vi "ReversedEngineering StateReverseDialog.vi"(5 "error in (no error)":errorcluster, 6 "NewDiagram":bool) -> (15 "StateDiagramReverseOptions":T5={"Clear All Current States"=FALSE, "UseMenuItem"=TRUE, "InsertArrayQueuedElementsVI"="", "Add Actions"=TRUE, "StateDiagramSerachActions"={"Action"=enum."OnlyTheseVIs", "VINames"=[], "LimitActions(VIs)"=0}, "AddCaseCommentsAsActions"=FALSE, "IgnoreStatesNotUsed"=FALSE, "CommentsSerachActions"={"MinimumTextLength"=0, "OnlyTopLeftComment"=FALSE, "CommentPrefix"=""}, "TransitionMode"=enum."Add to current transtion text", "ActionMode"=enum."Add to current action text"}, 16 "Cancel":bool, 19 "error out":errorcluster)   [LabVIEW 2012]
uses:
  <resource>/Framework/Providers/Open_GDS/UML/ReversedEngineering/private/ReversedEngineering StateDiagramReverseOptions.ctl
  <resource>/Framework/Providers/Open_GDS/UML/ReversedEngineering/private/ReversedEngineering StateDiagramSerachActions.ctl
  <resource>/Framework/Providers/Open_GDS/UML/ReversedEngineering/ReversedEngineering StateAnalyseVIAction.ctl
  <resource>/Framework/Providers/Open_GDS/UML/ReversedEngineering/private/ReversedEngineering StateDiagramCommentSearchType.ctl
  <resource>/Framework/Providers/Open_GDS/UML/UMLEditor/UMLEditor_StoredPathes.ctl
  <resource>/Framework/Providers/Open_GDS/UML/ContextHelp/ContextHelp_HelpTexts.ctl
  <resource>/Framework/Providers/Open_GDS/ClassProviders/Common/File/File_StoredPathesActions.ctl
panel:
  in  "ActionMode":T1(ring) caption="Action text"
  in  "TransitionMode":T2(ring) caption="Transition text"
  in  "CommentsSerachActions":T3
  in  "IgnoreStatesNotUsed":bool caption="Using Queued Based State Machines"
  in  "AddCaseCommentsAsActions":bool caption="Using Queued Based State Machines"
  in  "QueuedSettings":bool
  in  "UseQueuedStateMachines":bool caption="Using Queued Based State Machines"
  in  "Help":bool
  in  "SearchCriteria":T4={"NoOfAction"=10, "VI-List"=[], "VI-filter"=0, "ClearList"=FALSE, "AddVI"=FALSE, "AddVIs"=FALSE, "AddVIsRec"=FALSE} caption="Search for Actions(VIs)" {"VI-filter" items=["<Do not use VI-filter>", "Only allow VI-s found in the VI-List", "Allow all VIs except the ones in the VI-List"]; "NoOfAction" min=1 max=50}
  in  "SearchForVIs":bool
  in  "Cancel":bool
  in  "OK":bool
  in  "ClearStates":bool caption="Clear All Current States on the diagram"
  # "If the states should be search it checks all subvis and functions in every case."
  # "Select what actions(functions) that should be searched for. If the selected action exists in the state this action will be listed in the diagram."
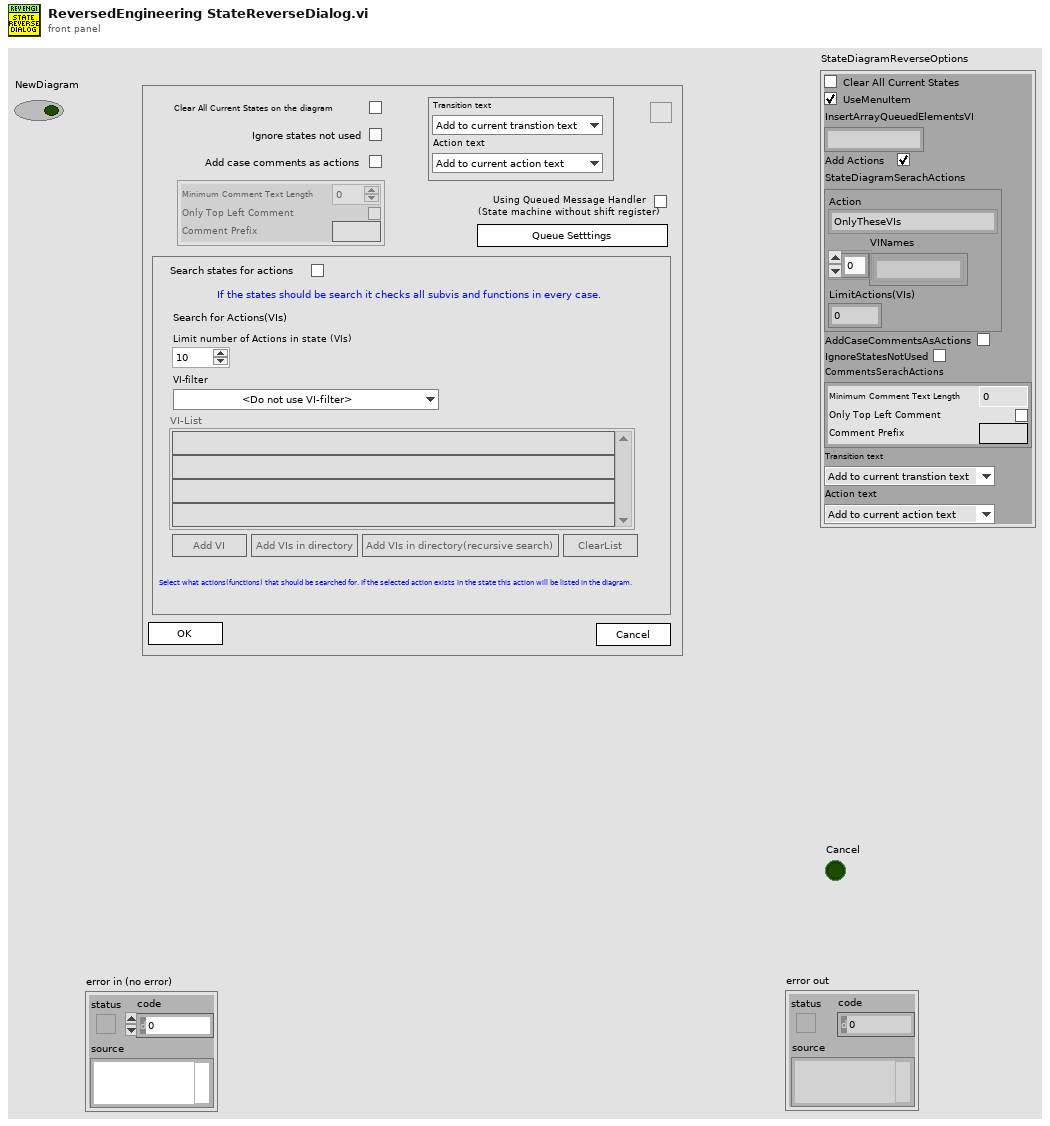
[diagram p1: front panel]
types:
  T1 = enum16{"Add to current action text", "Replace action text"}
  T2 = enum16{"Add to current transtion text", "Replace transition text"}
  T3 = typedef "ReversedEngineering StateDiagramCommentSearchType.ctl" = cluster{"MinimumTextLength":i32, "OnlyTopLeftComment":bool, "CommentPrefix":string}
  T4 = cluster{"NoOfAction":i32, "VI-List":string[], "VI-filter":u16, "ClearList":bool, "AddVI":bool, "AddVIs":bool, "AddVIsRec":bool}
  T5 = typedef "ReversedEngineering StateDiagramReverseOptions.ctl" = cluster{"Clear All Current States":bool, "UseMenuItem":bool, "InsertArrayQueuedElementsVI":string, "Add Actions":bool, "StateDiagramSerachActions":T6, "AddCaseCommentsAsActions":bool, "IgnoreStatesNotUsed":bool, "CommentsSerachActions":T3, "TransitionMode":enum16{"Add to current transtion text", "Replace transition text"}, "ActionMode":enum16{"Add to current action text", "Replace action text"}}
  T6 = typedef "ReversedEngineering StateDiagramSerachActions.ctl" = cluster{"Action":T7, "VINames":string[], "LimitActions(VIs)":i32}
  T7 = typedef "ReversedEngineering StateAnalyseVIAction.ctl" = enum16{"OnlyTheseVIs", "NotTheseVIs"}
  T8 = typedef "UMLEditor_StoredPathes.ctl" = enum16{"LastSearchPath", "QueuedArrayStateVI", "ClassBasePath", "ViTemplatePath", "ApplicationTemplatePath", "IniFilePath", "WizDir", "RevPlugInPath"}
  T9 = typedef "ContextHelp_HelpTexts.ctl" = enum16{"None(Hide)", "Default", "Help", "Welcome", "GettingStarted", "ClassDiagram_Help", "SequenceDiagram_Help", "UseCaseDiagram_Help", "BSelect", "BClass", "BInterface", "BPackage", "BNote", "BDependency", "BInheritance", "BInterfaceImplementation", "BAssociation", "BAggregation", "BCompAggregation", "BNoteConnector", "BObject", "BActionBar", "BCall", "BSystem", "BActor", "BUseCase", "BGeneralization", "BIncludes", "BExtends", "BUseCaseDiagramAssociation", "ClassRelationshipEdge editDialog_Bent Style", "ClassRelationshipEdge editDialog_RelationType", "ClassRelationshipEdge editDialog_Reverse association", "ClassRelationshipEdge editDialog_Start label", "ClassRelationshipEdge editDialog_Middle label", "ClassRelationshipEdge editDialog_End label", "UMLEditor reversedEngineering_Pathes", "ReversedEngineering StateReverseDialog_Help", "ReversedEngineering StateQueuedSettings_Help", "UMLEditor reversedEngineering_AddTopVIs", "UMLEditor reversedEngineering_AddClasses", "UMLEditor reversedEngineering_AddDirs", "UMLEditor reversedEngineering_Recursively", "UMLEditor reversedEngineering_Remove", "UMLEditor reversedEngineering_ClearList", "UMLEditor reversedEngineering_HideSubAss", "UMLEditor reversedEngineering_CreateTypes", "UMLEditor reversedEngineering_OnlyInheritance", "UMLEditor reversedEngineering_CreateApplication", "UMLEditor reversedEngineering_OK", "UMLEditor reversedEngineering_Cancel", "UMLEditor reversedEngineering_Help", "UMLEditor createWizardScriptFile_ScriptfilePath", "UMLEditor createWizardScriptFile_ClassPath", "UMLEditor createWizardScriptFile_Use", "UMLEditor createWizardScriptFile_PrivateDirName", "UMLEditor createWizardScriptFile_DirAppend", "UMLEditor createWizardScriptFile_Separator Character", "UMLEditor createWizardScriptFile_OK", "UMLEditor createWizardScriptFile_Cancel", "UMLEditor createWizardScriptFile_Help", "ClassNode editDialog_Class Name", "InterfaceNode editDialog_Class Name", "ClassNode editDialog_Attribute", "ClassNode editDialog_Methods", "InterfaceNode editDialog_Methods", "ClassNode editDialog_connection", "InterfaceNode editDialog_connection", "ClassNode editDialog_StereoType", "ClassNode editDialog_ShowAttrib", "ClassNode editDialog_ShowMethods", "ClassNode editDialog_ClassPath", "ClassNode editDialog_AddAttribute", "ClassNode editDialog_AddMethod", "InterfaceNode editDialog_AddMethod", "ClassNode AttributeGuide_AttributeName", "ClassNode AttributeGuide_Array?", "ClassNode AttributeGuide_Data Type", "ClassNode AttributeGuide_RefName", "ClassNode AttributeGuide_Preview", "ClassNode AttributeGuide_OK", "ClassNode AttributeGuide_Cancel", "ClassNode MethodGuide_Visibility", "ClassNode MethodGuide_Method Name", "ClassNode MethodGuide_Preview", "ClassNode MethodGuide_OK", "ClassNode MethodGuide_Cancel", "CallNode EditCallProperties_AllButtons", "ObjectNode EditObjectlProperties_AllButtons", "ActorNode EditActorProperties_AllButtons", "UseCaseRelationshipNode EditUseCaselProperties_AllButtons", "UseCaseNode EditUseCaselProperties_AllButtons", "SystemNode EditSystemProperties_AllButtons", "ReversedEngineering UpdateAttributes_AllButtons", "StateNode editDialog_AllButtons", "StateTransition editDialog_AllButtons", "ArrangeNodes Main_Picture", "ArrangeNodes Main_Zoom", "ArrangeNodes Main_Auto Zoom", "ArrangeNodes Main_shorten", "ArrangeNodes Main_Min Length", "ArrangeNodes Main_Max Length", "ArrangeNodes Main_increase", "ArrangeNodes Main_decrease", "ArrangeNodes Main_Shake", "ArrangeNodes Main", "BState", "BInitialState", "BFinalState", "BStateTransition", "StateDiagram_Help", "StateDiagram_PropertiesAllButtons", "ReversedEngineering StateReverseDialog_ClearStates", "ReversedEngineering StateReverseDialog_UseQueuedStateMachines", "ReversedEngineering StateReverseDialog_QueuedSettings", "ReversedEngineering StateReverseDialog_SearchForVIs", "ReversedEngineering StateReverseDialog_SearchCriteria", "OptionsDialog_ClassBasePath", "OptionsDialog_VIPath", "OptionsDialog_ApplicationPath", "OptionsDialog_WizDir", "OptionsDialog_IniFilePath", "OptionsDialog_DefineColors", "OptionsDialog_Help", "OptionsDialog_CreateTypes", "ClassRelationshipEdge editDialog_SplitWire"}
  T10 = typedef "File_StoredPathesActions.ctl" = enum16{"Get Path", "Set Path", "Delete Path", "Clear All Paths"}
  T11 = typedef "ContextHelp_ShowType.ctl" = cluster{"Header":string, "Picture":picture, "Text":string}
  T12 = enum32{"existing file", "new file", "new or existing file", "existing dir", "new dir", "new or existing dir", "existing file (use LLBs)", "new file (use LLBs)", "new or existing file (use LLBs)", "new or existing file or directory (use LLBs)"}
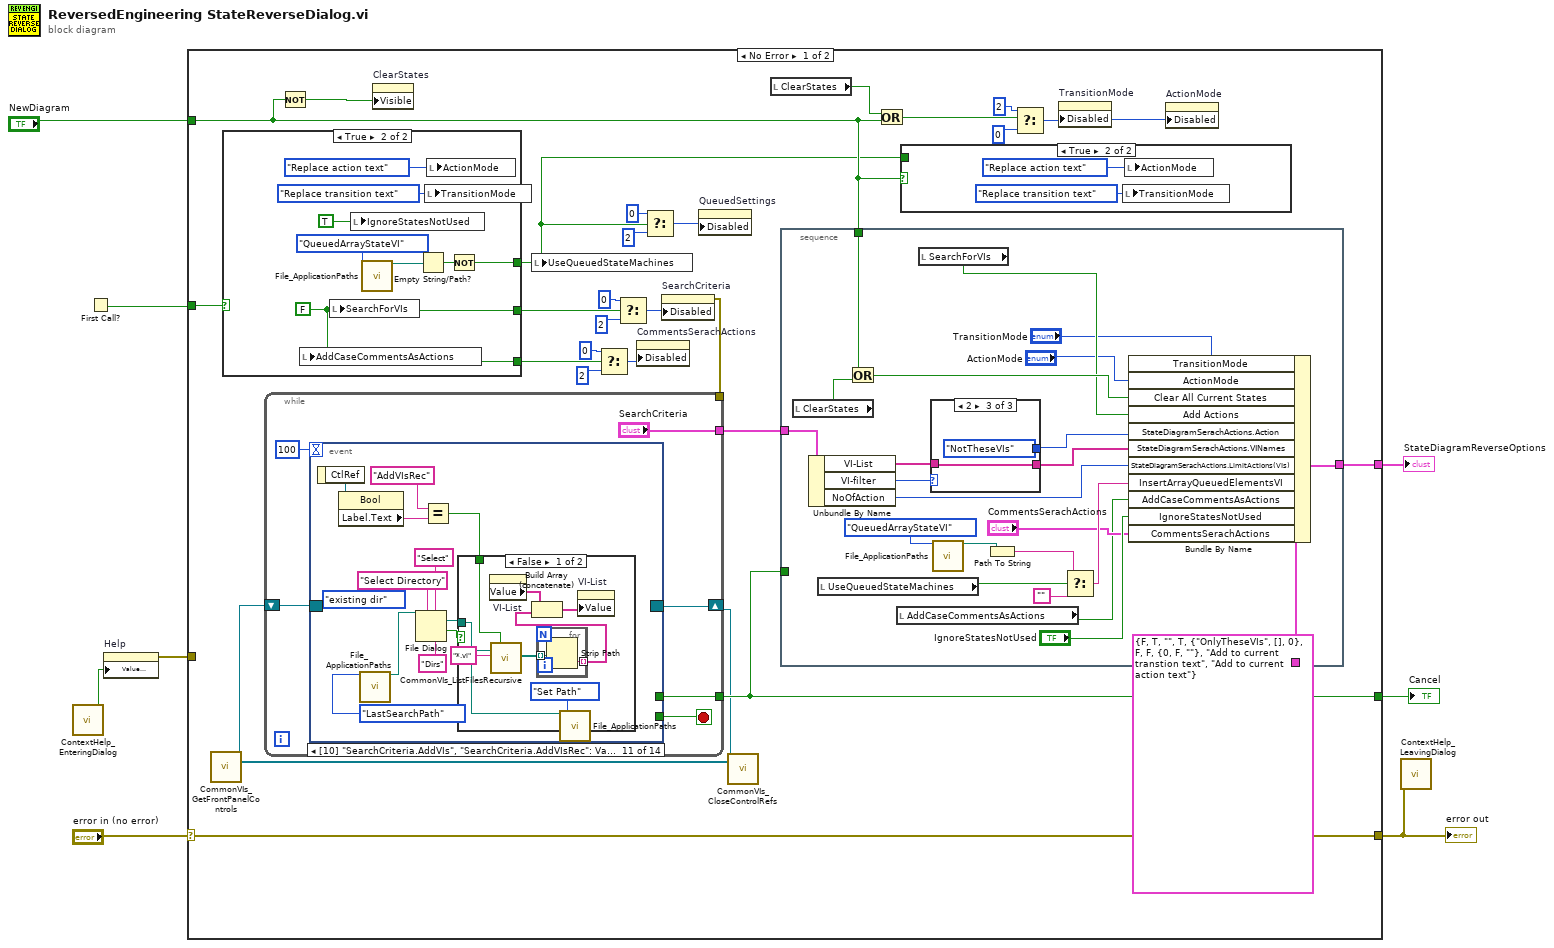
[diagram p0: block diagram]
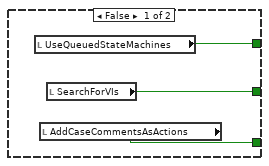
[diagram p3: hidden frame]
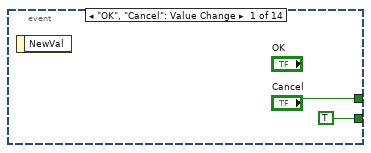
[diagram p4: hidden frame]
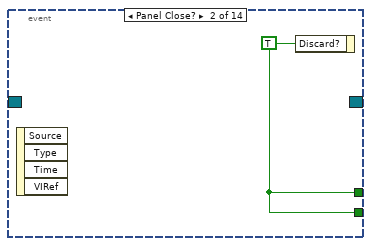
[diagram p5: hidden frame]
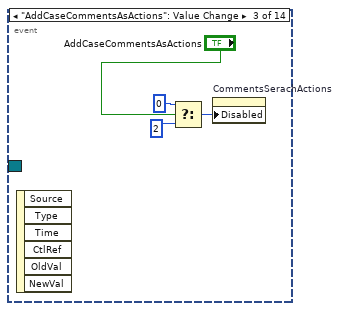
[diagram p6: hidden frame]
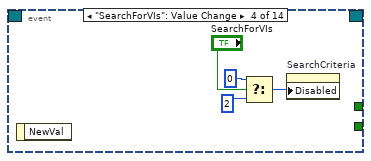
[diagram p7: hidden frame]
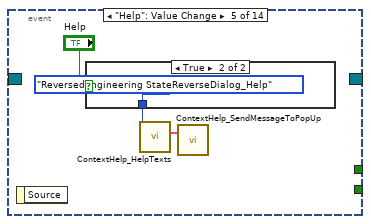
[diagram p8: hidden frame]
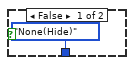
[diagram p9: hidden frame]
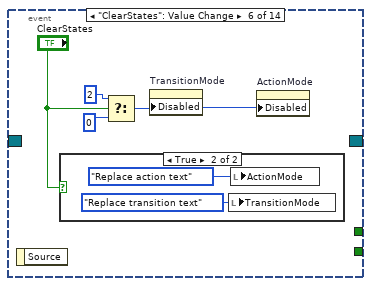
[diagram p10: hidden frame]
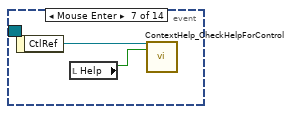
[diagram p12: hidden frame]
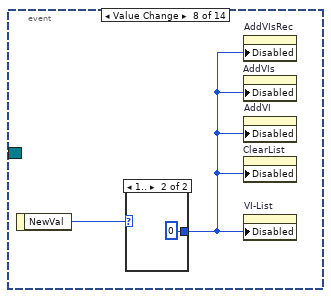
[diagram p13: hidden frame]
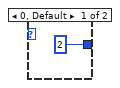
[diagram p14: hidden frame]
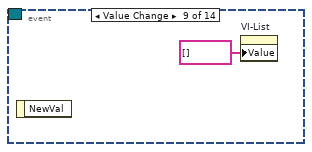
[diagram p15: hidden frame]
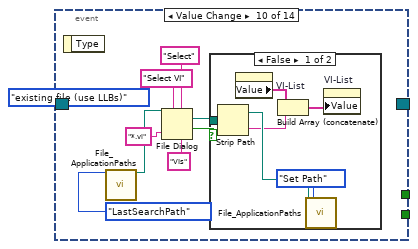
[diagram p16: hidden frame]
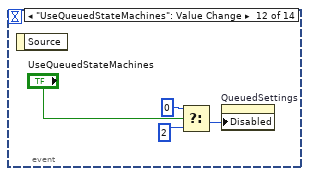
[diagram p19: hidden frame]
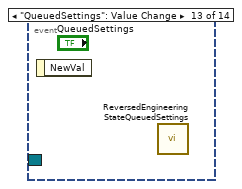
[diagram p20: hidden frame]
diagram:
  n1 = call <resource>:"ContextHelp_EnteringDialog.vi"() -> ("HelpStatus"=w4:bool)  [unwired: 1 in, 18 out]
  n2 = First Call?() -> (First Call?: T/F=w1:bool)
  n3 = property on="Help" class="Bool (strict)"("Value (Signaling)"=w4) -> (error out=w3:errorcluster)  [unwired: 2 in, 1 out]
  n4 = case shown="No Error" "error in (no error)" {
    selector: "error in (no error)" -> [w35 w155]
    tunnel: [w35 w155] -> w2
    tunnel: [w34 _] -> w7
    tunnel: [w36 _] -> w6
    tunnel: "NewDiagram" -> [w10 _]
    tunnel: w3 -> [_ _]
    tunnel: w1 -> [w27 _]
    frame No Error {
      n5 = call <resource>:"CommonVIs_GetFrontPanelControls.vi"() -> ("Event Registration Refnum"=w25:refnum<event-registration>, "ControlRefs"=w23:refnum<vi>[])  [unwired: 2 in, 16 out]
      n6 = case shown="True" w27 {
        tunnel: [w42 w46] -> w26
        tunnel: [w41 w47] -> w9
        tunnel: [w40 w46] -> w16
        frame False {
          n7 = local read "UseQueuedStateMachines"() -> (w41:bool)
          n8 = local read "AddCaseCommentsAsActions"() -> (w40:bool)
          n9 = local read "SearchForVIs"() -> (w42:bool)
        }
        frame True {
          w46 = FALSE ("SearchForVIs")
          n10 = local write "AddCaseCommentsAsActions"(w46) -> ()
          n11 = local write "SearchForVIs"(w46) -> ()
          n12 = local write "IgnoreStatesNotUsed"(TRUE ("IgnoreStatesNotUsed")) -> ()
          n13 = call <resource>:"File_ApplicationPaths.vi"("PathName"=UMLEditor_StoredPathes."QueuedArrayStateVI" ("UMLPathes")) -> ("Path Out"=w49:path)  [unwired: 3 in, 15 out]
          n14 = Empty String/Path?(string/path=w49) -> (empty?=w48:bool)
          n15 = local write "TransitionMode"(T2."Replace transition text" ("TransitionMode")) -> ()
          n16 = local write "ActionMode"(T1."Replace action text" ("ActionMode")) -> ()
          n17 = Not(x=w48) -> (.not. x?=w47:bool)
        }
      }
      n18 = Not(x=w10) -> (.not. x?=w29:bool)
      n19 = property on="ClearStates" class="Bool (strict)"("Visible"=w29) -> ()  [unwired: 2 in, 2 out]
      n20 = local write "UseQueuedStateMachines"(w9) -> ()
      n21 = Select(t=u8 0, s=w16, f=u8 2 ("Disabled")) -> (s? t:f=w17:u8)
      n22 = Select(t=u8 0, s=w26, f=u8 2 ("Disabled")) -> (s? t:f=w31:u8)
      n23 = property on="CommentsSerachActions" class="Clust (strict)"("Disabled"=w17) -> ()  [unwired: 2 in, 2 out]
      n24 = Select(t=u8 0, s=w9, f=u8 2 ("Disabled")) -> (s? t:f=w20:u8)
      n25 = property on="SearchCriteria" class="Clust"("Disabled"=w31) -> (error out=w30:errorcluster)  [unwired: 2 in, 1 out]
      n26 = while {
        tunnel: [w56] -> w34
        tunnel: w30 -> [_]
        tunnel: ["SearchCriteria"] -> w28
        shift-right: [w51] -> w24
        shift-left: w25 -> [w52]
        stop <- w55 stop-if-true
        n27 = event shown="[10] \"SearchCriteria.AddVIs\", \"SearchCriteria.AddVIsRec\": Value Change" {
          selector: w52 -> [_ _ _ _ _ _ _ _ _ _ _ _ _ _]
          dyn-events: [_ _ _ _ _ _ _ _ _ _ _ _ _ _] -> w51
          timeout: 100 -> [_ _ _ _ _ _ _ _ _ _ _ _ _ _]
          tunnel: ["Cancel" w59 _ _ _ _ _ _ _ _ _ _ _ _] -> w56
          tunnel: [TRUE w59 _ _ _ _ _ _ _ _ _ _ _ _] -> w55
          event "OK", "Cancel": Value Change {
            n28 = event-data() -> ()  [unwired: 2 out]
          }
          event Panel Close? {
            w59 = TRUE ("Discard?")
            n29 = event-data() -> ()  [unwired: 5 out]
            n30 = event-data("Discard?"=w59) -> ()  [unwired: 1 in, 1 out]
          }
          event "AddCaseCommentsAsActions": Value Change {
            n31 = event-data() -> ()  [unwired: 7 out]
            n32 = Select(t=u8 0, s="AddCaseCommentsAsActions", f=u8 2 ("Disabled")) -> (s? t:f=w63:u8)
            n33 = property on="CommentsSerachActions" class="Clust (strict)"("Disabled"=w63) -> ()  [unwired: 2 in, 2 out]
          }
          event "SearchForVIs": Value Change {
            n34 = event-data() -> ()  [unwired: 2 out]
            n35 = Select(t=u8 0, s="SearchForVIs", f=u8 2 ("Disabled")) -> (s? t:f=w65:u8)
            n36 = property on="SearchCriteria" class="Clust"("Disabled"=w65) -> ()  [unwired: 2 in, 2 out]
          }
          event "Help": Value Change {
            n37 = event-data() -> ()  [unwired: 2 out]
            n38 = case shown="True" "Help" {
              tunnel: [ContextHelp_HelpTexts."None(Hide)" ("HelpText") ContextHelp_HelpTexts."ReversedEngineering StateReverseDialog_Help" ("HelpText")] -> w69
              frame False {
              }
              frame True {
              }
            }
            n39 = call <resource>:"ContextHelp_HelpTexts.vi"("HelpText (enum or string)"=w69) -> ("HelpOut"=w70:T11)  [unwired: 18 out]
            n40 = call <resource>:"ContextHelp_SendMessageToPopUp.vi"("PopUpMessage"=w70) -> ()  [unwired: 2 in, 17 out]
          }
          event "ClearStates": Value Change {
            n41 = event-data() -> ()  [unwired: 2 out]
            n42 = case shown="True" "ClearStates" {
              frame False {
              }
              frame True {
                n43 = local write "TransitionMode"(T2."Replace transition text" ("TransitionMode")) -> ()
                n44 = local write "ActionMode"(T1."Replace action text" ("ActionMode")) -> ()
              }
            }
            n45 = Select(t=u8 2, s="ClearStates", f=u8 0 ("Disabled")) -> (s? t:f=w76:u8)
            n46 = property on="TransitionMode" class="Enum (strict)"("Disabled"=w76) -> ()  [unwired: 2 in, 2 out]
            n47 = property on="ActionMode" class="Enum (strict)"("Disabled"=w76) -> ()  [unwired: 2 in, 2 out]
          }
          event Mouse Enter {
            n48 = event-data() -> ("CtlRef"=w80:refnum<vi>)  [unwired: 1 out]
            n49 = local read "Help"() -> (w79:bool)
            n50 = call <resource>:"ContextHelp_CheckHelpForControl.vi"("Ctl Refnum"=w80, "Help"=w79) -> ()  [unwired: 1 in, 17 out]
          }
          event "SearchCriteria.VI-filter": Value Change {
            n51 = event-data() -> ("NewVal"=w82:u16)  [unwired: 1 out]
            n52 = case shown="1.." w82 {
              tunnel: [u8 2 ("Disabled") u8 0 ("Disabled")] -> w81
              frame 0, Default {
              }
              frame 1.. {
              }
            }
            n53 = property on="AddVIsRec" class="Bool"("Disabled"=w81) -> ()  [unwired: 2 in, 2 out]
            n54 = property on="AddVIs" class="Bool"("Disabled"=w81) -> ()  [unwired: 2 in, 2 out]
            n55 = property on="AddVI" class="Bool"("Disabled"=w81) -> ()  [unwired: 2 in, 2 out]
            n56 = property on="ClearList" class="Bool"("Disabled"=w81) -> ()  [unwired: 2 in, 2 out]
            n57 = property on="VI-List" class="Arr (strict)"("Disabled"=w81) -> ()  [unwired: 2 in, 2 out]
          }
          event "SearchCriteria.ClearList": Value Change {
            n58 = event-data() -> ()  [unwired: 2 out]
            n59 = property on="VI-List" class="Arr (strict)"("Value"=string[] []) -> ()  [unwired: 2 in, 2 out]
          }
          event "SearchCriteria.AddVI": Value Change {
            (unwired) T12."existing file (use LLBs)" ("select mode (2)")
            n60 = event-data() -> ()  [unwired: 2 out]
            n61 = call <resource>:"File_ApplicationPaths.vi"("PathName"=UMLEditor_StoredPathes."LastSearchPath" ("UMLPathes")) -> ("Path Out"=w91:path)  [unwired: 3 in, 15 out]
            n62 = File Dialog(4:"VIs" ("pattern label"), 5:"Select" ("button label"), 6:"*.vi" ("pattern"), 7:"Select VI" ("prompt"), 11:w91) -> (1:w86:bool, 3:w90:path)  [unwired: 1 in, 3 out]
            n63 = case shown="False" w86 {
              tunnel: w90 -> [w98 _]
              frame False {
                n64 = Strip Path(path=w98) -> (stripped path=w97:path, name=w95:string)
                n65 = property on="VI-List" class="Arr (strict)"() -> ("Value"=w96:string[])  [unwired: 2 in, 2 out]
                n66 = Build Array (concatenate)(w96, w95) -> (w94:string[])
                n67 = call <resource>:"File_ApplicationPaths.vi"("Path In"=w97, "Method (Get Path)"=File_StoredPathesActions."Set Path") -> ()  [unwired: 2 in, 16 out]
                n68 = property on="VI-List" class="Arr (strict)"("Value"=w94) -> ()  [unwired: 2 in, 2 out]
              }
              frame True {
              }
            }
          }
          event "SearchCriteria.AddVIs", "SearchCriteria.AddVIsRec": Value Change {
            (unwired) T12."existing dir" ("select mode (2)")
            n69 = event-data() -> ("CtlRef"=w103:refnum<vi>)  [unwired: 1 out]
            n70 = property class="Bool"(reference=w103) -> ("Label.Text"=w102:string)  [unwired: 1 in, 2 out]
            n71 = call <resource>:"File_ApplicationPaths.vi"("PathName"=UMLEditor_StoredPathes."LastSearchPath" ("UMLPathes")) -> ("Path Out"=w108:path)  [unwired: 3 in, 15 out]
            n72 = File Dialog(4:"Dirs" ("pattern label"), 5:"Select" ("button label"), 7:"Select Directory" ("prompt"), 11:w108) -> (1:w104:bool, 3:w107:path)  [unwired: 1 in, 4 out]
            n73 = Equal?(x="AddVIsRec", y=w102) -> (x = y?=w100:bool)
            n74 = case shown="False" w104 {
              tunnel: w107 -> [w114 _]
              tunnel: w100 -> [w111 _]
              frame False {
                n75 = property on="VI-List" class="Arr (strict)"() -> ("Value"=w117:string[])  [unwired: 2 in, 2 out]
                n76 = call <resource>:"CommonVIs_ListFilesRecursive.vi"("directory path"=w114, "FileSearchPattern"="*.vi", "RecusiveSearch(True)"=w111) -> ("Files"=w113:path[])  [unwired: 3 in, 13 out]
                n77 = for {
                  tunnel: w113 -> [w120] mode=indexing
                  tunnel: [w119] -> w112 mode=indexing
                  n78 = Strip Path(path=w120) -> (name=w119:string)  [unwired: 1 out]
                }
                n79 = Build Array (concatenate)(w117, w112) -> (w116:string[])
                n80 = call <resource>:"File_ApplicationPaths.vi"("PathName"=w114, "Method (Get Path)"=File_StoredPathesActions."Set Path") -> ()  [unwired: 2 in, 16 out]
                n81 = property on="VI-List" class="Arr (strict)"("Value"=w116) -> ()  [unwired: 2 in, 2 out]
              }
              frame True {
              }
            }
          }
          event "UseQueuedStateMachines": Value Change {
            n82 = event-data() -> ()  [unwired: 2 out]
            n83 = Select(t=u8 0, s="UseQueuedStateMachines", f=u8 2 ("Disabled")) -> (s? t:f=w122:u8)
            n84 = property on="QueuedSettings" class="Bool"("Disabled"=w122) -> ()  [unwired: 2 in, 2 out]
          }
          event "QueuedSettings": Value Change {
            n85 = event-data() -> ()  [unwired: 2 out]
            n86 = call <resource>:"ReversedEngineering StateQueuedSettings.vi"() -> ()  [unwired: 1 in, 19 out]
          }
          event Timeout {
            n87 = event-data() -> ()  [unwired: 4 out]
            n88 = property class="VI"("Front Panel Window:Is Frontmost"=TRUE ("Front Panel Window:Open")) -> ()  [unwired: 2 in, 2 out]
          }
        }
      }
      n89 = property on="QueuedSettings" class="Bool"("Disabled"=w20) -> ()  [unwired: 2 in, 2 out]
      n90 = call <resource>:"CommonVIs_CloseControlRefs.vi"("Event Registration Refnum"=w24, "ControlRefs"=w23) -> ()  [unwired: 1 in, 17 out]
      n91 = local read "ClearStates"() -> (w13:bool)
      n92 = stacked-sequence {
        tunnel: T5 {"Clear All Current States"=FALSE, "UseMenuItem"=TRUE, "InsertArrayQueuedElementsVI"="", "Add Actions"=TRUE, "StateDiagramSerachActions"={"Action"=enum."OnlyTheseVIs", "VINames"=[], "LimitActions(VIs)"=0}, "AddCaseCommentsAsActions"=FALSE, "IgnoreStatesNotUsed"=FALSE, "CommentsSerachActions"={"MinimumTextLength"=0, "OnlyTopLeftComment"=FALSE, "CommentPrefix"=""}, "TransitionMode"=enum."Add to current transtion text", "ActionMode"=enum."Add to current action text"} ("StateDiagramReverseOptions") -> [w148]
        tunnel: [w140] -> w36
        tunnel: w34 -> [_]
        tunnel: w10 -> [w146]
        tunnel: w28 -> [w139]
        frame #0 {
          n93 = local read "ClearStates"() -> (w128:bool)
          n94 = Unbundle By Name(w139) -> ("VI-List"=w144:string[], "VI-filter"=w145:u16, "NoOfAction"=w142:i32)
          n95 = local read "UseQueuedStateMachines"() -> (w137:bool)
          n96 = Or(x=w146, y=w128) -> (x .or. y?=w147:bool)
          n97 = local read "AddCaseCommentsAsActions"() -> (w129:bool)
          n98 = local read "SearchForVIs"() -> (w141:bool)
          n99 = case shown="2" w145 {
            tunnel: w144 -> [_ w151 w153]
            tunnel: [string[] [] ("VI-List") w151 w153] -> w143
            tunnel: [ReversedEngineering_StateAnalyseVIAction."NotTheseVIs" ("StateDiagramSerachActions.Action") ReversedEngineering_StateAnalyseVIAction."OnlyTheseVIs" ("StateDiagramSerachActions.Action") ReversedEngineering_StateAnalyseVIAction."NotTheseVIs" ("StateDiagramSerachActions.Action")] -> w138
            frame 0, Default {
            }
            frame 1 {
            }
            frame 2 {
            }
          }
          n100 = call <resource>:"File_ApplicationPaths.vi"("PathName"=UMLEditor_StoredPathes."QueuedArrayStateVI" ("UMLPathes")) -> ("Path Out"=w133:path)  [unwired: 3 in, 15 out]
          n101 = Path To String(path=w133) -> (string=w132:string)
          n102 = Select(t=w132, s=w137, f="") -> (s? t:f=w136:string)
          n103 = Bundle By Name(cluster=w148, "TransitionMode"="TransitionMode", "ActionMode"="ActionMode", "Clear All Current States"=w147, "Add Actions"=w141, "StateDiagramSerachActions.Action"=w138, "StateDiagramSerachActions.VINames"=w143, "StateDiagramSerachActions.LimitActions(VIs)"=w142, "InsertArrayQueuedElementsVI"=w136, "AddCaseCommentsAsActions"=w129, "IgnoreStatesNotUsed"="IgnoreStatesNotUsed", "CommentsSerachActions"="CommentsSerachActions") -> (w140:T5)
        }
      }
      n104 = Or(x=w13, y=w10) -> (x .or. y?=w12:bool)
      n105 = case shown="True" w10 {
        tunnel: w9 -> [_ _]
        frame False {
        }
        frame True {
          n106 = local write "TransitionMode"(T2."Replace transition text" ("TransitionMode")) -> ()
          n107 = local write "ActionMode"(T1."Replace action text" ("ActionMode")) -> ()
        }
      }
      n108 = Select(t=u8 2, s=w12, f=u8 0 ("Disabled")) -> (s? t:f=w11:u8)
      n109 = property on="TransitionMode" class="Enum (strict)"("Disabled"=w11) -> ()  [unwired: 2 in, 2 out]
      n110 = property on="ActionMode" class="Enum (strict)"("Disabled"=w11) -> ()  [unwired: 2 in, 2 out]
    }
    frame Error {
    }
  }
  "error out" <- w2
  "Cancel" <- w7
  "StateDiagramReverseOptions" <- w6
  n111 = call <resource>:"ContextHelp_LeavingDialog.vi"("error in (no error)"=w2) -> ()  [unwired: 19 out]
